vi "CPU_MEM_references.vi"() -> ()   [LabVIEW 2018]
panel:
  in  "CHAR ROM":refnum<data-value>
  in  "BASIC ROM":refnum<data-value>
  in  "KERNAL ROM":refnum<data-value>
  out "video mem":refnum<data-value>
  in  "Color mem ref":refnum<data-value>
  in  "SID mem ref":refnum<data-value>
  in  "RAM ref":refnum<data-value>
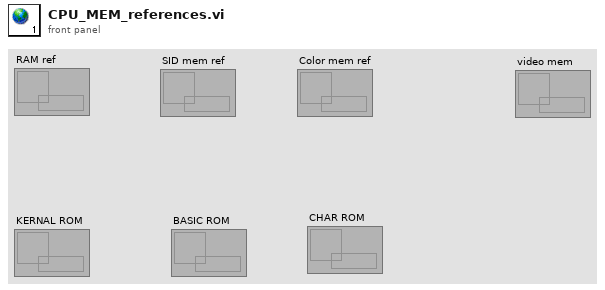
[diagram p1: front panel]
diagram:
